vi "Calculate T0.vi"(10 "Waveform":waveform(dbl), 11 "Data In":dbl[](array[numeric])) -> (1 "Data Out T0":timestamp, 2 "dt":dbl, 3 "Data Out":dbl[](array[numeric]))   [LabVIEW 2024, in "FFT.lvlib" / "FFT.lvclass"]
uses:
  FFT.lvclass
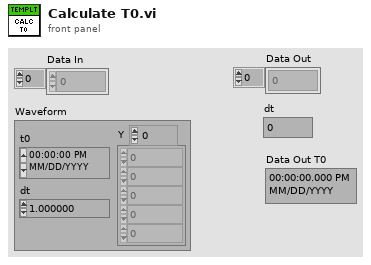
[diagram p1: front panel]
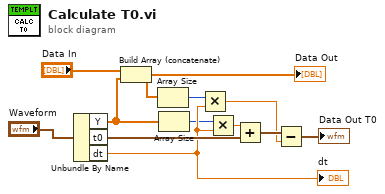
[diagram p0: block diagram]
diagram:
  n1 = Unbundle By Name("Waveform") -> ("Y"=w10:dbl[], "t0"=w8:timestamp, "dt"=w3:dbl)
  "dt" <- w3
  n2 = Build Array (concatenate)("Data In", w10) -> (w6:dbl[])
  "Data Out" <- w6
  n3 = Array Size(array=w6) -> (size(s)=w1:i32)
  n4 = Array Size(array=w10) -> (size(s)=w2:i32)
  n5 = Multiply(x=w1, y=w3) -> (x*y=w5:dbl)
  n6 = Multiply(x=w2, y=w3) -> (x*y=w9:dbl)
  n7 = Add(x=w9, y=w8) -> (x+y=w7:timestamp)
  n8 = Subtract(x=w7, y=w5) -> (x-y=→"Data Out T0":timestamp)
